vi "Acquire-images.vi"(8 "error in":errorcluster, 10 "UI ref. in":refnum<data-value>, 11 "Data ref. in":refnum<data-value>) -> (0 "error IO":errorcluster, 2 "UI ref.":refnum<data-value>, 3 "Data ref.":refnum<data-value>)   [LabVIEW 2013, in "CameraVision.lvlib" / "CV-Main.lvclass"]
uses:
  CV-Main.lvclass
  UI/CV-UI.lvclass
  UI/Module-states.ctl
  UI/CV-UI.lvclass/CV-UI.ctl
  CV-Main.lvclass/CV-Main.ctl
  UI/Notifier-with-memory-timeStamp.vi
  UI/Read Acquisition.vi
  UI/Read Acquire stop.vi
  Read Acquis params.vi
  Read Buffers.vi
  Read Config params.vi
  Acquisition/CV-Acquisition.lvclass
  Buffers/CV-Buffers.lvclass
  Configuration/CV-Configuration.lvclass
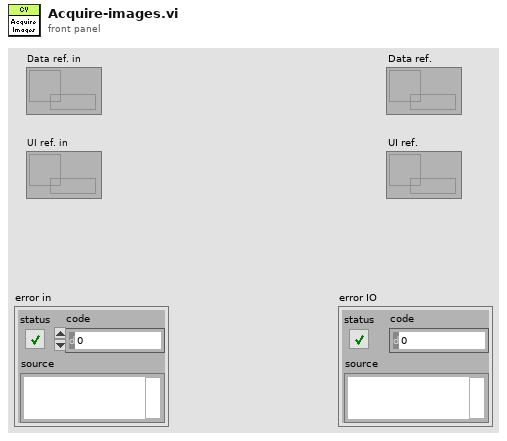
[diagram p1: front panel]
types:
  T1 = typedef "CameraVision.lvlib/CV-UI.lvclass/Module-states.ctl" = enum16{"Inactive", "Active", "Data-loss", "Error", "Simulation", "Synchronizing", "Initialized", "Released"}
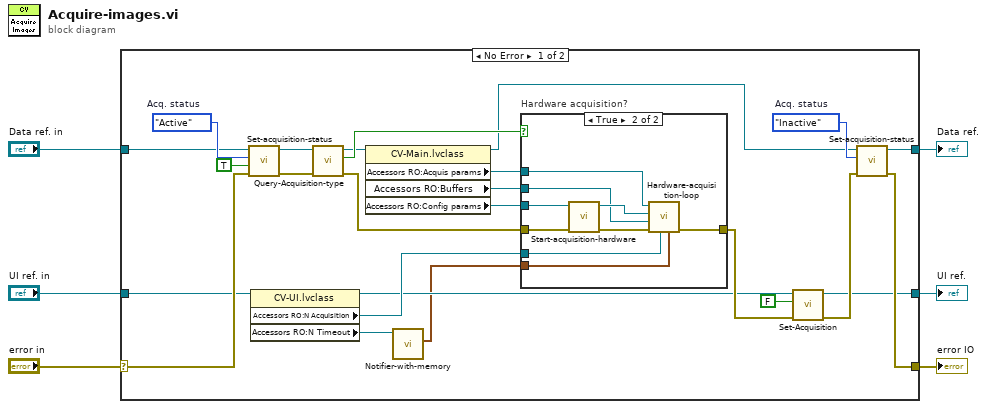
[diagram p0: block diagram]
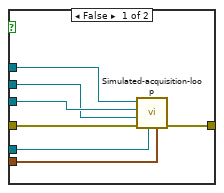
[diagram p2: hidden frame]
diagram:
  n1 = case shown="No Error" "error in" {
    selector: "error in" -> [w10 w50]
    tunnel: [w18 w50] -> w6
    tunnel: "UI ref. in" -> [w9 w49]
    tunnel: "Data ref. in" -> [w28 w48]
    tunnel: [w13 w49] -> w1
    tunnel: [w19 w48] -> w2
    frame No Error {
      w31 = Module-states."Inactive"  # Acq. status
      w30 = Module-states."Active"  # Acq. status
      n2 = call "Set-acquisition-status.vi"("error in"=w10, "Reset errors?"=TRUE, "Acq. status in"=w30, "Data ref. in"=w28) -> ("error IO"=w26:errorcluster, "Data ref."=w27:refnum<data-value>)  [unwired: 5 in, 1 out]
      n3 = property class="CV-UI.lvclass"(reference=w9) -> (reference out=w14:refnum<data-value>, "Accessors RO:N Acquisition"=w22:refnum<notifier>, "Accessors RO:N Timeout"=w8:refnum<notifier>)  [unwired: 1 in, 1 out]
      n4 = call "Query-Acquisition-type.vi"("error in"=w26, "Data ref. in"=w27) -> ("error IO"=w21:errorcluster, "Hardware acquisiton?"=w29:bool, "Data ref."=w25:refnum<data-value>)  [unwired: 7 in]
      n5 = property class="CV-Main.lvclass"(reference=w25) -> (reference out=w20:refnum<data-value>, "Accessors RO:Acquis params"=w24:refnum<data-value>, "Accessors RO:Buffers"=w11:refnum<class "CV-Buffers.lvclass">, "Accessors RO:Config params"=w23:refnum<data-value>)  [unwired: 1 in, 1 out]
      n6 = call-poly "Notifier-with-memory.vi"("Notifier in"=w8) -> ("Notification"=w7:timestamp)  [unwired: 9 in, 1 out]
      n7 = case "Hardware acquisition?" shown="True" w29 {
        tunnel: w24 -> [w38 w45]
        tunnel: w23 -> [w35 w47]
        tunnel: w22 -> [w33 w40]
        tunnel: w21 -> [w37 w44]
        tunnel: [w36 w42] -> w16
        tunnel: w11 -> [w34 w41]
        tunnel: w7 -> [w32 w39]
        frame False {
          n8 = call "Simulated-acquisition-loop.vi"("Timeout"=w32, "Acquisition notif"=w33, "error in (no error)"=w37, "Buffers"=w34, "Config. params. ref. in"=w35, "Acquis. params. ref. in"=w38) -> ("error out"=w36:errorcluster)  [unwired: 3 in, 2 out]
        }
        frame True {
          n9 = call "Start-acquisition-hardware.vi"("error in"=w44, "Config. params in"=w47) -> ("error IO"=w43:errorcluster, "Config. params"=w46:refnum<data-value>)  [unwired: 8 in]
          n10 = call "Hardware-acquisition-loop.vi"("Timeout"=w39, "Acquisition notif"=w40, "error in (no error)"=w43, "Buffers"=w41, "Config. params. ref. in"=w46, "Acquis. params. ref. in"=w45) -> ("error out"=w42:errorcluster)  [unwired: 3 in, 2 out]
        }
      }
      n11 = call "Set-Acquisition.vi"("error in (no error)"=w16, "Acquisition"=FALSE ("Stop"), "UI ref. in"=w14) -> ("error out"=w15:errorcluster, "UI ref."=w13:refnum<data-value>)  [unwired: 7 in]
      n12 = call "Set-acquisition-status.vi"("error in"=w15, "Acq. status in"=w31, "Data ref. in"=w20) -> ("error IO"=w18:errorcluster, "Data ref."=w19:refnum<data-value>)  [unwired: 6 in, 1 out]
    }
    frame Error {
    }
  }
  "error IO" <- w6
  "Data ref." <- w2
  "UI ref." <- w1
